vi "Commit Hardware Relay State.vi"(0 "DevicePropertyRelay in":refnum<class "DevicePropertyRelay.lvclass">, 5 "Session Handle":T1, 11 "error in (no error)":errorcluster) -> (4 "DevicePropertyRelay out":refnum<class "DevicePropertyRelay.lvclass">, 15 "error out":errorcluster)   [LabVIEW 2015, in "SLSC Switch.lvlib" / "DevicePropertyRelay.lvclass"]
uses:
  DevicePropertyRelay.lvclass
  SLSC Session/Typedefs/Session Handle.ctl
  SLSC Session/SLSC Session.lvclass
  DevicePropertyRelay.lvclass/DevicePropertyRelay.ctl
  Relay Interface/RelayInterface.lvclass
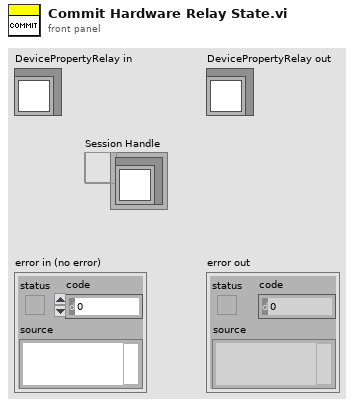
[diagram p1: front panel]
types:
  T1 = typedef "SLSC Switch.lvlib/SLSC Session.lvclass/Session Handle.ctl" = refnum<data-value>
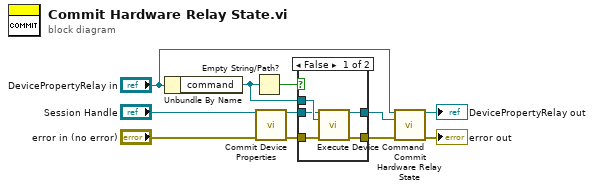
[diagram p0: block diagram]
diagram:
  n1 = Unbundle By Name("DevicePropertyRelay in") -> ("command"=w11:refnum<k21>)
  n2 = Empty String/Path?(string/path=w11) -> (empty?=w10:bool)
  n3 = call "Commit Device Properties.vi"("Session Handle in"="Session Handle", "error in (no error)"="error in (no error)") -> ("Session Handle out"=w2:T1, "error out"=w3:errorcluster)  [unwired: 12 in]
  n4 = case shown="False" w10 {
    tunnel: w11 -> [w16 _]
    tunnel: w3 -> [w14 w18]
    tunnel: [w13 w18] -> w9
    tunnel: w2 -> [w15 w17]
    tunnel: [w12 w17] -> w1
    frame False {
      n5 = call "Execute Device Command.vi"("Session Handle in"=w15, "command"=w16, "error in (no error)"=w14) -> ("Session Handle out"=w12:T1, "error out"=w13:errorcluster)  [unwired: 11 in]
    }
    frame True {
    }
  }
  n6 = call-parent "Commit Hardware Relay State.vi"("RelayInterface in"="DevicePropertyRelay in", "Session Handle in"=w1, "error in (no error)"=w9) -> ("RelayInterface out"=→"DevicePropertyRelay out":refnum<class "DevicePropertyRelay.lvclass">, "error out"=→"error out":errorcluster)  [unwired: 11 in]
